vi "Wfm skaluj ramke.vi"(7 "Plot Area Widths":u32[](array[numeric]), 8 "error in (no error)":errorcluster, 11 "Wfm Refs in":refnum<vi>[](array[refnum])) -> (0 "error out":errorcluster, 3 "Wfm Refs out":refnum<vi>[](array[refnum]))   [LabVIEW 2014]
doc: "Skaluje szerokoœæ ramki wykresu dla wszystkich podpiêtych komponentów\nwzglêdem pierwszego z dwóch najmniejszych"
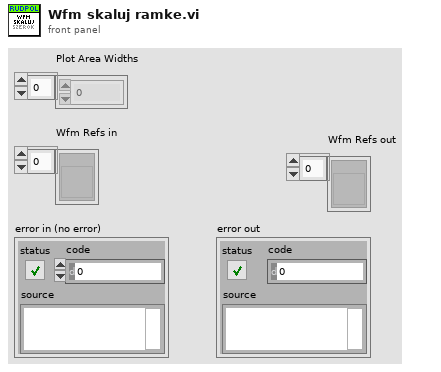
[diagram p1: front panel]
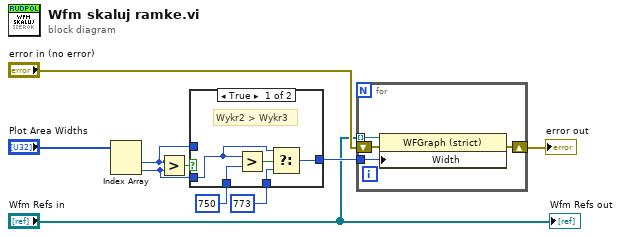
[diagram p0: block diagram]
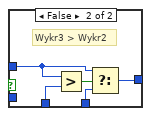
[diagram p2: hidden frame]
diagram:
  n1 = Index Array(array="Plot Area Widths") -> (element #1=w4:u32, element #2=w5:u32)  [unwired: 2 in]
  n2 = Greater?(x=w4, y=w5) -> (0:w3:bool)
  n3 = case shown="True" w3 {
    tunnel: w4 -> [_ w19]
    tunnel: w5 -> [w14 _]
    tunnel: u32 773 ("y") -> [w12 w18]
    tunnel: u32 750 ("y") -> [w13 w17]
    tunnel: [w11 w16] -> w8
    frame True {
      # "Wykr2 > Wykr3"
      n4 = Greater?(x=w14, y=w13) -> (0:w15:bool)
      n5 = Select(t=w14, s=w15, f=w12) -> (s? t:f=w11:u32)
    }
    frame False {
      # "Wykr3 > Wykr2"
      n6 = Greater?(x=w19, y=w17) -> (0:w20:bool)
      n7 = Select(t=w19, s=w20, f=w18) -> (s? t:f=w16:u32)
    }
  }
  n8 = for {
    tunnel: "Wfm Refs in" -> [w24] mode=indexing
    tunnel: w8 -> [w23]
    shift-right: [w21] -> w10
    shift-left: "error in (no error)" -> [w22]
    n9 = property class="WFGraph (strict)"(reference=w24, error in=w22, "Width"=w23) -> (error out=w21:errorcluster)  [unwired: 1 out]
  }
  "error out" <- w10
  "Wfm Refs out" <- "Wfm Refs in"
